vi "DynamixelSimple.vi"() -> ()   [LabVIEW 2018]
uses:
  <userlib>/dxl_x86_c/dxl_x86_c.lvlib
panel:
  in  "stop":bool
  out "Present Position":dbl(knob) scale=0.0..360.0
  in  "Goal Position":dbl(knob) scale=0.0..360.0
  in  "Ring":u16(ring) items=["Please Select", "Current Control", "Velocity", "Position", "Extended Position", "Current-based Position Control"]
  out "function return":i32
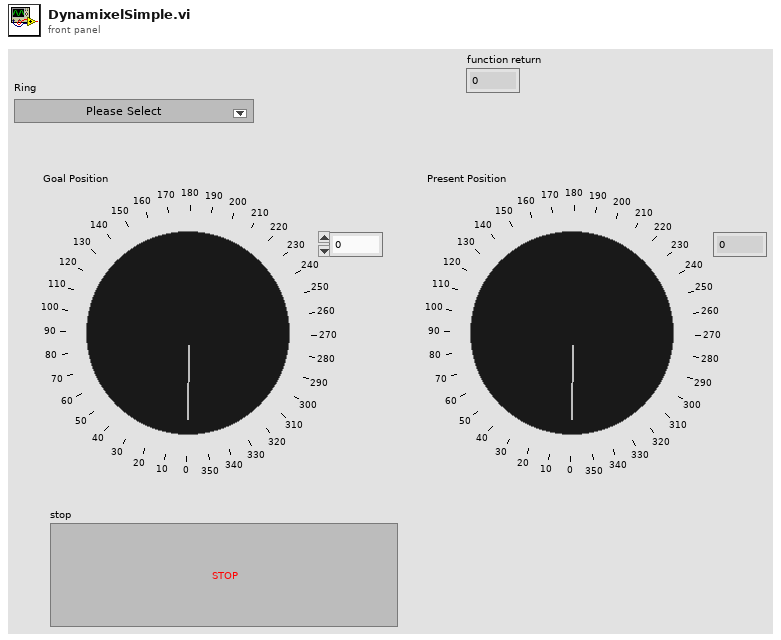
[diagram p1: front panel]
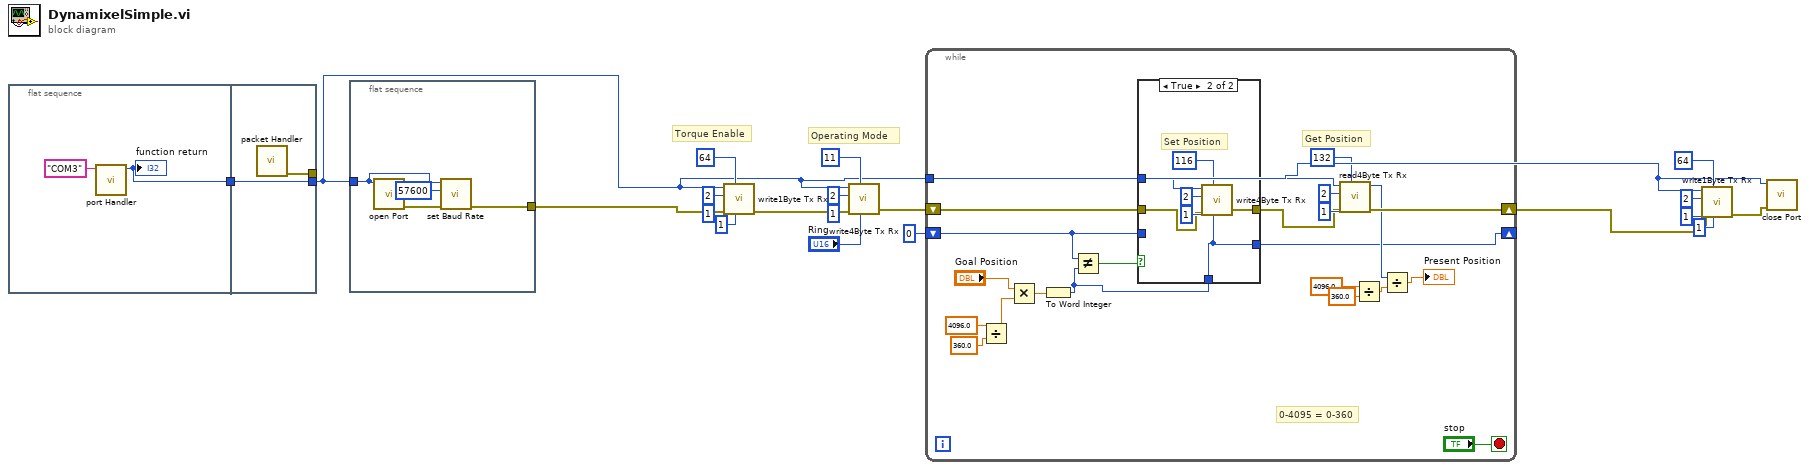
[diagram p0: block diagram]
diagram:
  # "Operating Mode"
  # "Torque Enable"
  n1 = flat-sequence {
    tunnel: [w21] -> w20
    tunnel: [w24] -> w4
    tunnel: w20 -> [w24]
    tunnel: [w23] -> _
    frame #0 {
      n2 = call <userlib>:"port Handler.vi"("port_name"="COM3") -> ("function return"=w21:i32)  [unwired: 9 in, 1 out]
      "function return" <- w21
    }
    frame #1 {
      n3 = call <userlib>:"packet Handler.vi"() -> ("error out"=w23:errorcluster)  [unwired: 11 in]
    }
  }
  n4 = flat-sequence {
    tunnel: w4 -> [w28]
    tunnel: [w26] -> w19
    frame #0 {
      n5 = call <userlib>:"open Port.vi"("port_num"=w28) -> ("error out"=w27:errorcluster)  [unwired: 9 in, 1 out]
      n6 = call <userlib>:"set Baud Rate.vi"("error in (no error)"=w27, "baudrate"=57600, "port_num"=w28) -> ("error out"=w26:errorcluster)  [unwired: 7 in, 1 out]
    }
  }
  n7 = call <userlib>:"write1Byte Tx Rx.vi"("data"=u32 1, "address"=u16 64, "error in (no error)"=w19, "id"=u8 1, "protocol_version"=2, "port_num"=w4) -> ("error out"=w14:errorcluster)  [unwired: 5 in]
  n8 = call <userlib>:"write4Byte Tx Rx.vi"("data"="Ring", "address"=u16 11, "error in (no error)"=w14, "id"=u8 1, "protocol_version"=2, "port_num"=w4) -> ("error out"=w9:errorcluster)  [unwired: 5 in]
  n9 = while {
    tunnel: w4 -> [w45]
    shift-right: [w44] -> w2
    shift-left: w9 -> [w50]
    shift-right: [w35] -> _
    shift-left: u32 0 ("milliseconds to wait") -> [w37]
    stop <- "stop" stop-if-true
    # "Get Position"
    # "0-4095 = 0-360"
    n10 = Divide(x=4096.0 ("y"), y=360.0 ("x")) -> (x/y=w31:dbl)
    n11 = Multiply(x="Goal Position", y=w31) -> (x*y=w39:dbl)
    n12 = To Word Integer(number=w39) -> (16bit integer=w34:i16)
    n13 = Not Equal?(x=w37, y=w34) -> (x != y?=w36:bool)
    n14 = case shown="True" w36 {
      tunnel: w50 -> [w52 w56]
      tunnel: [w52 w55] -> w46
      tunnel: w45 -> [_ w54]
      tunnel: w37 -> [w51 _]
      tunnel: [w51 w53] -> w35
      tunnel: w34 -> [_ w53]
      frame False {
      }
      frame True {
        # "Set Position"
        n15 = call <userlib>:"write4Byte Tx Rx.vi"("data"=w53, "address"=u16 116, "error in (no error)"=w56, "id"=u8 1, "protocol_version"=2, "port_num"=w54) -> ("error out"=w55:errorcluster)  [unwired: 5 in]
      }
    }
    n16 = call <userlib>:"read4Byte Tx Rx.vi"("address"=u16 132, "error in (no error)"=w46, "id"=u8 1, "protocol_version"=2, "port_num"=w45) -> ("error out"=w44:errorcluster, "function return"=w40:u32)  [unwired: 5 in]
    n17 = Divide(x=4096.0, y=360.0) -> (x/y=w43:dbl)
    n18 = Divide(x=w40, y=w43) -> (x/y=→"Present Position":dbl)
  }
  n19 = call <userlib>:"write1Byte Tx Rx.vi"("data"=u32 1, "address"=u16 64, "error in (no error)"=w2, "id"=u8 1, "protocol_version"=2, "port_num"=w4) -> ("error out"=w3:errorcluster)  [unwired: 5 in]
  n20 = call <userlib>:"close Port.vi"("error in (no error)"=w3, "port_num"=w4) -> ()  [unwired: 9 in, 1 out]
